vi "UnzipBook.vi"(2 "FileZipped":string, 4 "Parameters":T1={"Book Folder Name"="", "Full file name"="", "Remote Path"="bookfiles/", "Shelf folder"=path "", "Existing books"=[], "Dialog?"=enum."No Dialog", "New Format?"=FALSE}) -> (0 "error out":errorcluster, 1 "Book":path)   [LabVIEW 2012]
uses:
  <vilib>/zip/NI_Unzip.lvlib
  <userlib>/BotSpeak/Devices/EvalRIO/FTPCodes/FTPParameters.ctl
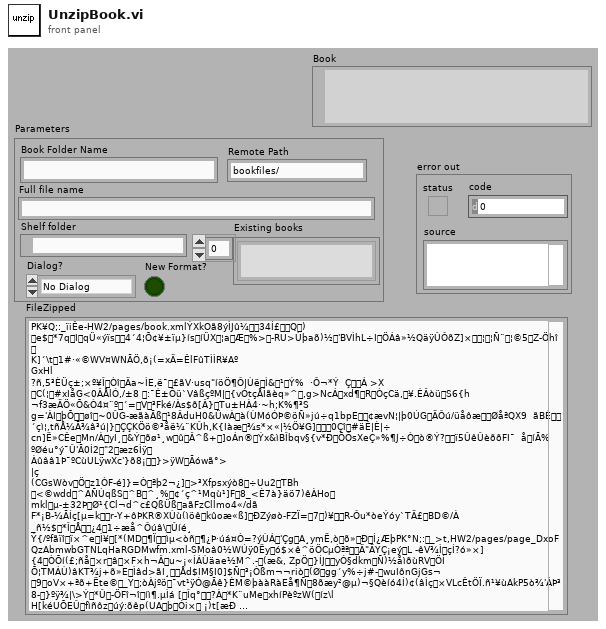
[diagram p1: front panel]
types:
  T1 = typedef "FTPParameters.ctl" = cluster{"Book Folder Name":string, "Full file name":string, "Remote Path":string, "Shelf folder":path, "Existing books":string[], "Dialog?":enum16{"No Dialog", "Dialog", "Overwrite"}, "New Format?":bool}
  T2 = enum16{"open", "replace", "create", "open or create", "replace or create", "replace or create with confirmation"}
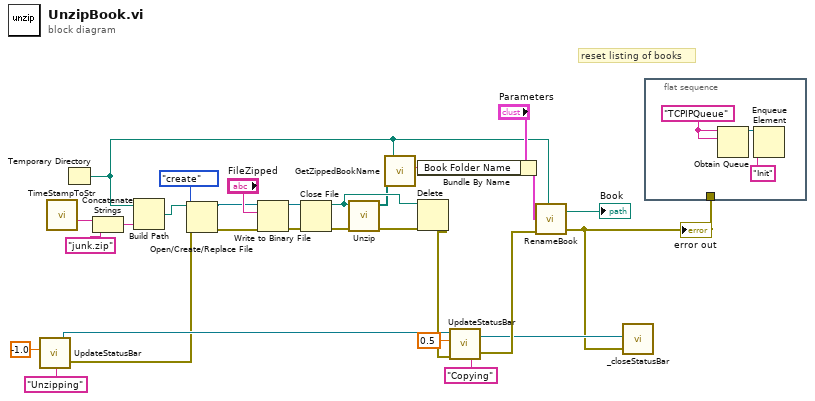
[diagram p0: block diagram]
diagram:
  # "reset listing of books"
  n1 = call <userlib>:"UpdateStatusBar.vi"("i"=-1.0, "Label"="Unzipping") -> ("reference out"=w8:refnum<vi>, "error out"=w5:errorcluster)  [unwired: 3 in]
  n2 = call <userlib>:"TimeStampToStr.vi"() -> ("date/time string"=w22:string)
  n3 = Temporary Directory() -> (w1:path)
  n4 = Concatenate Strings(w22, "junk.zip" ("Remote Path")) -> (w24:string)
  n5 = Build Path(base path=w1, name or relative path=w24) -> (appended path=w21:path)
  n6 = Open/Create/Replace File(file path (use dialog)=w21, error in=w5, operation (0:open)=T2."create") -> (refnum out=w18:refnum<file>, error out=w17:errorcluster)  [unwired: 4 out]
  n7 = Write to Binary File(file (use dialog)=w18, data="FileZipped", error in=w17) -> (refnum out=w19:refnum<file>, error out=w20:errorcluster)  [unwired: 4 out]
  n8 = Close File(refnum=w19, error in=w20) -> (path=w27:path, error out=w26:errorcluster)
  n9 = call <vilib>:"Unzip.vi"("error in (no error)"=w26, "Zip file"=w27) -> ("error out"=w28:errorcluster, "Unzipped files"=w15:path[])  [unwired: 2 in, 6 out]
  n10 = call <userlib>:"GetZippedBookName.vi"("Unzipped files"=w15, "path"=w1) -> ("String"=w3:string)
  n11 = Bundle By Name(cluster="Parameters", "Book Folder Name"=w3) -> (w2:T1)
  n12 = Delete(path (use dialog)=w27, error in=w28) -> (error out=w10:errorcluster)  [unwired: 5 out]
  n13 = call <userlib>:"UpdateStatusBar.vi"("reference in"=w8, "i"=0.5, "error in (no error)"=w10, "Label"="Copying") -> ("reference out"=w7:refnum<vi>, "error out"=w9:errorcluster)  [unwired: 1 in]
  n14 = call <userlib>:"RenameBook.vi"("Parameters"=w2, "base path"=w1, "error in"=w9) -> ("error out"=w6:errorcluster, "destination"=→"Book":path)  [unwired: 3 in]
  "error out" <- w6
  n15 = call <userlib>:"_closeStatusBar.vi"("error in (no error)"=w6, "reference out"=w7) -> ()  [unwired: 2 out]
  n16 = flat-sequence {
    tunnel: w6 -> [_]
    frame #0 {
      w31 = "TCPIPQueue" ("name (unnamed)")
      n17 = Obtain Queue(name (unnamed)=w31, element data type=w31) -> (queue out=w32:refnum<queue>)  [unwired: 3 in, 2 out]
      n18 = Enqueue Element(queue=w32, element="Init" ("name (unnamed)")) -> ()  [unwired: 2 in, 3 out]
    }
  }
